vi "Body Pane Resized-Event.vi"(8 "error in (no error)":errorcluster, 9 "NewBnds":T1, 10 "OldBnds":T1, 11 "Recipe Window in":refnum<class "Recipe Window.lvclass">) -> (0 "error out":errorcluster, 3 "Recipe Window out":refnum<class "Recipe Window.lvclass">)   [LabVIEW 2021, in "Recipe.lvlib" / "Recipe Window.lvclass"]
uses:
  Recipe Window.lvclass
  <vilib>/Utility/miscctls.llb/LVRectTypeDef.ctl
  Recipe Window.lvclass/Recipe Window.ctl
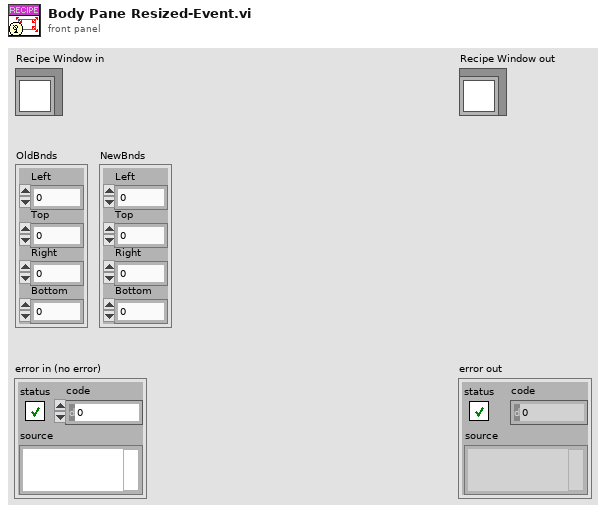
[diagram p1: front panel]
types:
  T1 = typedef "LVRectTypeDef.ctl" = cluster{"Left":i16, "Top":i16, "Right":i16, "Bottom":i16}
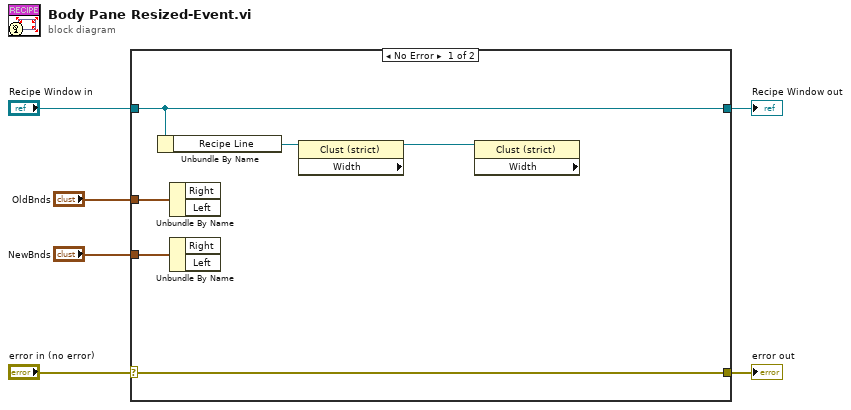
[diagram p0: block diagram]
diagram:
  n1 = case shown="No Error" "error in (no error)" {
    selector: "error in (no error)" -> [w12 w14]
    tunnel: [w12 w14] -> w5
    tunnel: [w11 w13] -> w3
    tunnel: "Recipe Window in" -> [w11 w13]
    tunnel: "OldBnds" -> [w8 _]
    tunnel: "NewBnds" -> [w7 _]
    frame No Error {
      n2 = Unbundle By Name(w11) -> ("Recipe Line"=w10:refnum<vi>)
      n3 = Unbundle By Name(w8) -> ()  [unwired: 2 out]
      n4 = Unbundle By Name(w7) -> ()  [unwired: 2 out]
      n5 = property class="Clust (strict)" props=["Width"](reference=w10) -> (reference out=w9:refnum<vi>)  [unwired: 1 in, 2 out]
      n6 = property class="Clust (strict)" props=["Width"](reference=w9) -> ()  [unwired: 1 in, 3 out]
    }
    frame Error {
    }
  }
  "error out" <- w5
  "Recipe Window out" <- w3
